vi "new line to operation.vi"(8 "error in":errorcluster, 10 "new line item":T1, 11 "Actual Configuration":refnum<class "Scan Engine configuration.lvclass">) -> (0 "error out":errorcluster, 1 "channel":refnum<class "TBM channel.lvclass">, 2 "Tag reference":refnum<class "tag descriptor.lvclass">, 3 "Scan Engine configuration out":refnum<class "Scan Engine configuration.lvclass">, 5 "new mapping?":bool)   [LabVIEW 2013, in "Scan Engine editor node.lvclass"]
uses:
  Scan Engine editor node.lvclass
  table line.ctl
  <vilib>/NI/Tag Bus Module Framework/channel/TBM channel.lvclass
  module/configuration/Scan Engine configuration.lvclass
  <vilib>/NI/Tag Bus/tag/tag descriptor.lvclass
  <vilib>/NI/Tag Bus/tag/tag descriptor.lvclass/tag descriptor.ctl
  <vilib>/NI/Tag Bus/tag/write tag name.vi
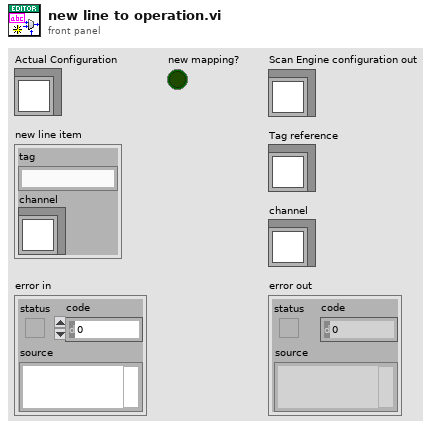
[diagram p1: front panel]
types:
  T1 = typedef "Scan Engine editor node.lvclass/table line.ctl" = cluster{"tag":string, "channel":refnum<class "TBM channel.lvclass">}
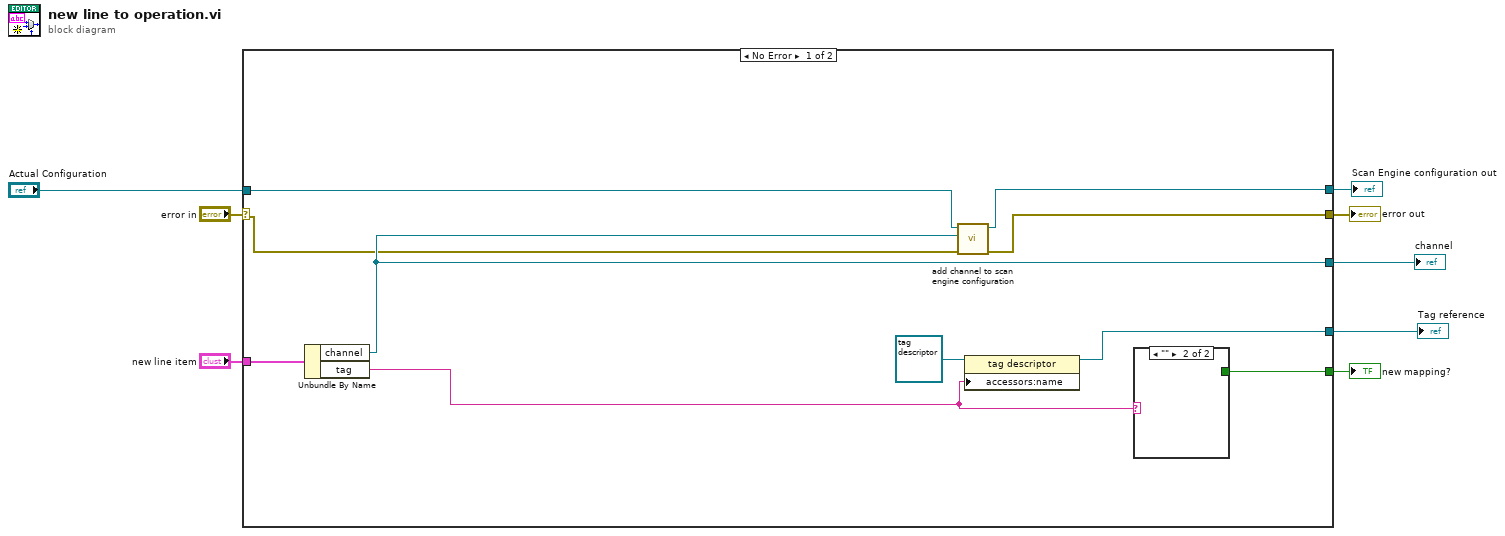
[diagram p0: block diagram]
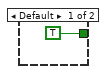
[diagram p2: hidden frame]
diagram:
  n1 = case shown="No Error" "error in" {
    selector: "error in" -> [w9 w21]
    tunnel: "new line item" -> [w18 _]
    tunnel: [w15 w21] -> w7
    tunnel: [w17 _] -> w5
    tunnel: "Actual Configuration" -> [w14 w20]
    tunnel: [w13 w20] -> w3
    tunnel: [w16 _] -> w2
    tunnel: [w10 _] -> w1
    frame No Error {
      n2 = Unbundle By Name(w18) -> ("channel"=w16:refnum<class "TBM channel.lvclass">, "tag"=w11:string)
      n3 = call "add channel to scan engine configuration.vi"("error in"=w9, "channel"=w16, "Scan Engine configuration in"=w14) -> ("error out"=w15:errorcluster, "Scan Engine configuration out"=w13:refnum<class "Scan Engine configuration.lvclass">)  [unwired: 7 in]
      n4 = property class="tag descriptor"(reference=refnum<class "tag descriptor.lvclass"> refnum ("tag"), "accessors:name"=w11) -> (reference out=w10:refnum<class "tag descriptor.lvclass">)  [unwired: 1 in, 1 out]
      n5 = case shown="\"\"" w11 {
        tunnel: [TRUE _] -> w17
        frame Default {
        }
        frame "" {
        }
      }
    }
    frame Error {
    }
  }
  "error out" <- w7
  "new mapping?" <- w5
  "Scan Engine configuration out" <- w3
  "channel" <- w2
  "Tag reference" <- w1
